vi "OxyGen_C02Scrub Calc.vi"(9 "Diagnostic Data In":bool[][](array[boolean]), 10 "Calculation Select":T1) -> (2 "Oxy Gen/C02 Scrub Rating Out":u32)   [LabVIEW 2020]
uses:
  Calculation Select_ENUM.ctl
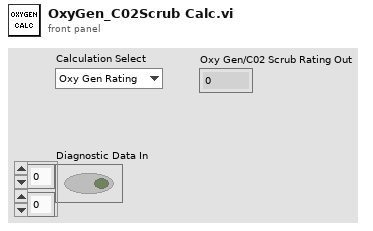
[diagram p1: front panel]
types:
  T1 = typedef "Calculation Select_ENUM.ctl" = enum16{"Oxy Gen Rating", "C02 Scrub Rating"}
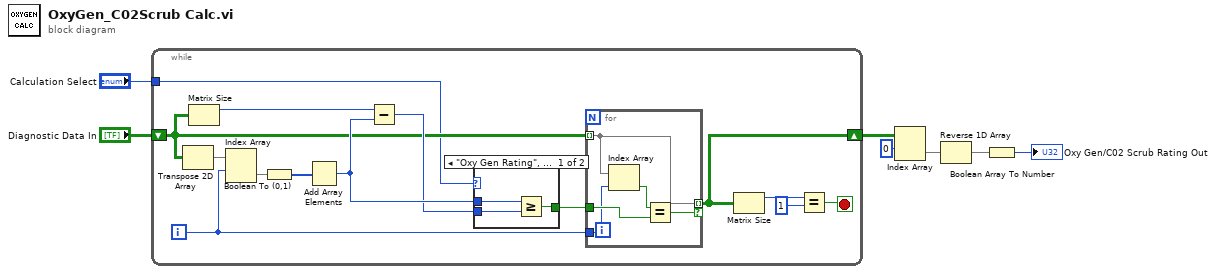
[diagram p0: block diagram]
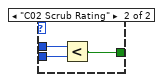
[diagram p2: hidden frame]
diagram:
  n1 = while {
    shift-right: [w12] -> w2
    shift-left: "Diagnostic Data In" -> [w10]
    tunnel: "Calculation Select" -> [w9]
    i -> [w15]
    stop <- w13 stop-if-true
    n2 = Transpose 2D Array(2D array=w10) -> (transposed array=w14:bool[][])
    n3 = Matrix Size(0:w10) -> (1:w11:i32)  [unwired: 1 out]
    n4 = Index Array(array=w14, index (row)=w15) -> (element=w18:bool[])  [unwired: 1 in]
    n5 = Boolean To (0,1)(Boolean=w18) -> (0, 1=w19:i16[])
    n6 = Add Array Elements(numeric array=w19) -> (sum=w21:i16)
    n7 = Subtract(x=w11, y=w21) -> (x-y=w20:i32)
    n8 = case shown="\"Oxy Gen Rating\", Default" w9 {
      tunnel: w21 -> [w24 w26]
      tunnel: w20 -> [w23 w27]
      tunnel: [w22 w25] -> w8
      frame "Oxy Gen Rating", Default {
        n9 = Greater Or Equal?(x=w24, y=w23) -> (x >= y?=w22:bool)
      }
      frame "C02 Scrub Rating" {
        n10 = Less?(x=w26, y=w27) -> (x < y?=w25:bool)
      }
    }
    n11 = for {
      tunnel: w8 -> [w32]
      tunnel: [w28] -> w12 mode=indexing if=w31
      tunnel: w15 -> [w30]
      tunnel: w10 -> [w28] mode=indexing
      n12 = Index Array(array=w28, index=w30) -> (element=w29:bool)
      n13 = Equal?(x=w29, y=w32) -> (x = y?=w31:bool)
    }
    n14 = Matrix Size(0:w12) -> (1:w17:i32)  [unwired: 1 out]
    n15 = Equal?(x=w17, y=1) -> (x = y?=w13:bool)
  }
  n16 = Index Array(array=w2, index (row)=0) -> (element=w4:bool[])  [unwired: 1 in]
  n17 = Reverse 1D Array(array=w4) -> (reversed array=w5:bool[])
  n18 = Boolean Array To Number(Boolean array=w5) -> (number=→"Oxy Gen/C02 Scrub Rating Out":u32)
